vi "Log Data.vi"(6 "Samples to Save In":u32, 8 "error in (no error)":errorcluster, 9 "Data":waveform(dbl)[](array[waveform]), 10 "Piezo Data":T1, 11 "Logging Configuration":T2) -> (0 "error out":errorcluster, 4 "Samples to Save Out":u32)   [LabVIEW 2013, in "Logging.lvlib"]
doc: "Use the Write To Measurement File Express VI to log data to disk in a LVM file."
uses:
  Logging.lvlib
  Logging Configuration.ctl
  Piezo/Piezo display.ctl
  <vilib>/Waveform/WDTOps.llb/WDT Index Channel DBL.vi
  Desktop/Simon Labview/Piezo.lvlib
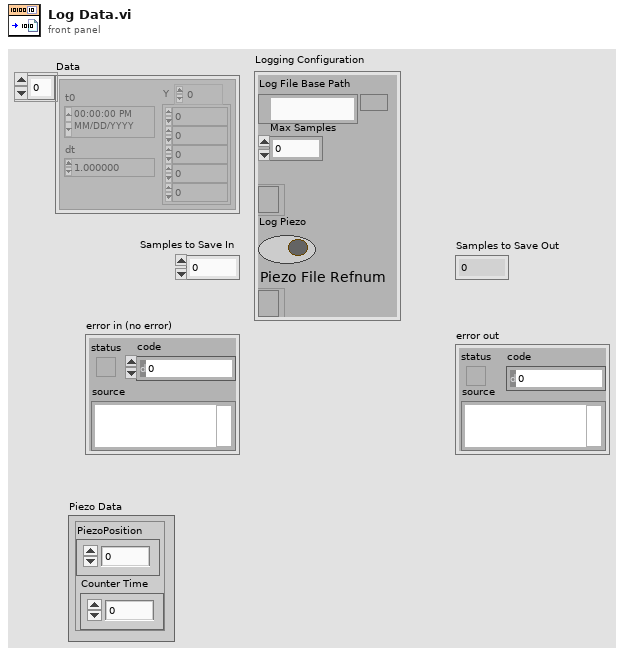
[diagram p1: front panel]
types:
  T1 = typedef "Piezo.lvlib/Piezo display.ctl" = cluster{"PiezoPosition":sgl, "Counter Time":i32}
  T2 = typedef "Logging.lvlib/Logging Configuration.ctl" = cluster{"Log File Base Path":path, "Max Samples":u32, "File Refnum":refnum<file>, "Log Piezo":bool, "Piezo File Refnum":refnum<file>}
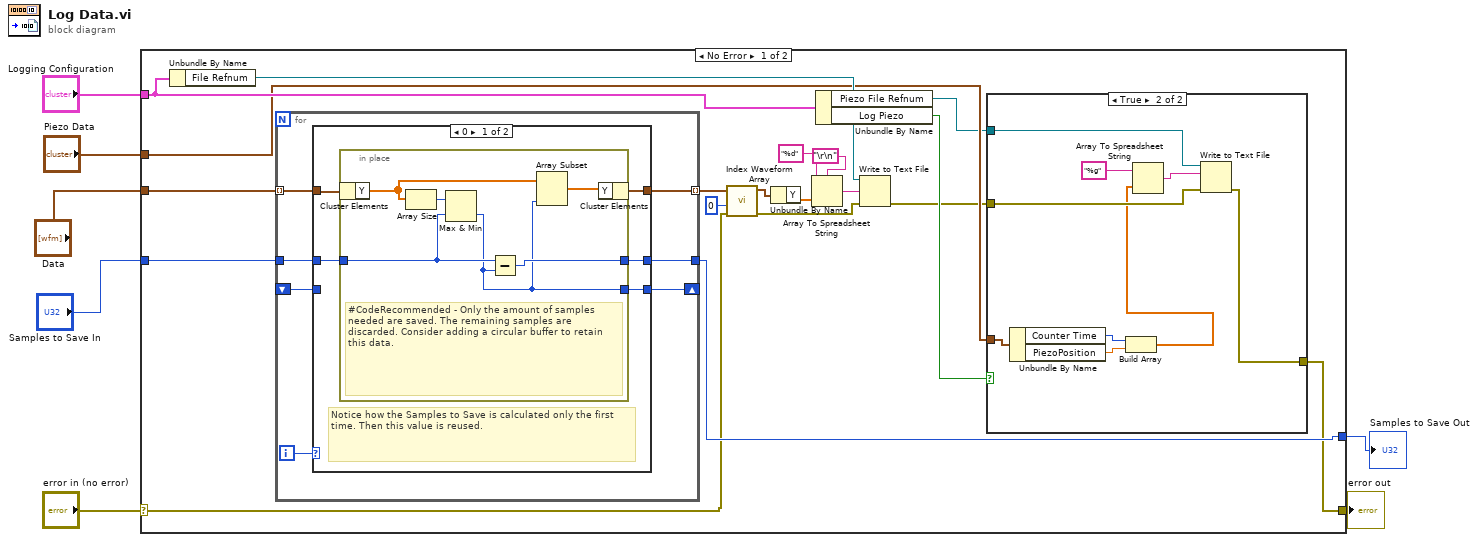
[diagram p0: block diagram]
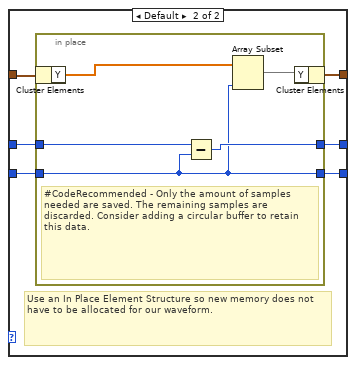
[diagram p3: hidden frame]
diagram:
  n1 = case shown="No Error" "error in (no error)" {
    selector: "error in (no error)" -> [w18 w67]
    tunnel: "Logging Configuration" -> [w13 _]
    tunnel: "Data" -> [w26 _]
    tunnel: [w8 w67] -> w6
    tunnel: "Samples to Save In" -> [w25 w66]
    tunnel: [w24 w66] -> w2
    tunnel: "Piezo Data" -> [w11 _]
    frame No Error {
      n2 = Unbundle By Name(w13) -> ("File Refnum"=w23:refnum<file>)
      n3 = for {
        tunnel: w26 -> [w42] mode=indexing
        tunnel: w25 -> [w43]
        tunnel: [w41] -> w21 mode=indexing
        tunnel: [w40] -> w24
        shift-right: [w38] -> _
        shift-left: _ -> [w37]
        i -> [w39]
        n4 = case shown="0" w39 {
          tunnel: w43 -> [w48 w60]
          tunnel: w42 -> [w44 w56]
          tunnel: [w45 w55] -> w41
          tunnel: [w47 w59] -> w40
          tunnel: [w46 w57] -> w38
          tunnel: w37 -> [_ w58]
          frame 0 {
            # "Notice how the Samples to Save is calculated only the first time. Then this value is reused."
            n5 = in-place {
              in-place-border: w48 -> [w53]
              in-place-border: [w52] -> w47
              in-place-border: [w49] -> w46
              # "#CodeRecommended - Only the amount of samples needed are saved. The remaining samples are discarded. Consider adding a circular buffer to retain this data."
              n6 = in-place-cluster #1(w44) -> ("Y"=w51:dbl[])
              n7 = Array Size(array=w51) -> (size(s)=w54:i32)
              n8 = Max & Min(x=w54, y=w53) -> (min(x,y)=w49:u32)  [unwired: 1 out]
              n9 = Subtract(x=w53, y=w49) -> (x-y=w52:u32)
              n10 = Array Subset(array=w51, length=w49) -> (w50:dbl[])  [unwired: 1 in]
              n11 = in-place-cluster #1("Y"=w50) -> (w45:waveform(dbl))
            }
          }
          frame Default {
            # "Use an In Place Element Structure so new memory does not have to be allocated for our waveform."
            n12 = in-place {
              in-place-border: w60 -> [w65]
              in-place-border: [w64] -> w59
              in-place-border: [w61] -> w57
              in-place-border: w58 -> [w61]
              # "#CodeRecommended - Only the amount of samples needed are saved. The remaining samples are discarded. Consider adding a circular buffer to retain this data."
              n13 = in-place-cluster #2(w56) -> ("Y"=w63:dbl[])
              n14 = Subtract(x=w65, y=w61) -> (x-y=w64:u32)
              n15 = Array Subset(array=w63, length=w61) -> (w62:dbl[])  [unwired: 1 in]
              n16 = in-place-cluster #2("Y"=w62) -> (w55:waveform(dbl))
            }
          }
        }
      }
      n17 = call-poly <vilib>:"Index Waveform Array.vi"("error in (no error)"=w18, "index"=0, "waveform array"=w21) -> ("error out"=w19:errorcluster, "waveform"=w17:waveform(dbl))  [unwired: 7 in]
      n18 = Unbundle By Name(w17) -> ("Y"=w16:dbl[])
      n19 = Array To Spreadsheet String(delimiter (Tab)="\r\n", array=w16, 3:"%d" ("format string")) -> (spreadsheet string=w22:string)
      n20 = Unbundle By Name(w13) -> ("Piezo File Refnum"=w10:refnum<file>, "Log Piezo"=w12:bool)
      n21 = Write to Text File(file (use dialog)=w23, text=w22, error in=w19) -> (error out=w9:errorcluster)  [unwired: 1 in, 2 out]
      n22 = case shown="True" w12 {
        tunnel: w11 -> [_ w34]
        tunnel: w10 -> [_ w36]
        tunnel: w9 -> [w27 w30]
        tunnel: [w27 w29] -> w8
        frame False {
        }
        frame True {
          n23 = Unbundle By Name(w34) -> ("Counter Time"=w33:i32, "PiezoPosition"=w32:sgl)
          n24 = Build Array(w33, w32) -> (w28:sgl[])
          n25 = Array To Spreadsheet String(array=w28, 3:"%g" ("format string")) -> (spreadsheet string=w35:string)  [unwired: 1 in]
          n26 = Write to Text File(file (use dialog)=w36, text=w35, error in=w30) -> (error out=w29:errorcluster)  [unwired: 1 in, 2 out]
        }
      }
    }
    frame Error {
    }
  }
  "error out" <- w6
  "Samples to Save Out" <- w2
